vi "Do.vi"(8 "error in (no error)":errorcluster, 10 "Actor in":refnum<class "Actor.lvclass">, 11 "SetInputChannels Msg":refnum<class "SetInputChannels Msg.lvclass">) -> (0 "error out":errorcluster, 2 "Actor out":refnum<class "Actor.lvclass">)   [LabVIEW 2023, in "Multiharp.lvlib" / "SetInputChannels Msg.lvclass"]
doc: "This VI delivers the message to the actor by calling the appropriate method(s) on the actor."
uses:
  SetInputChannels Msg.lvclass
  SetInputChannels Msg.lvclass/SetInputChannels Msg.ctl
  bbf59504-f208-437b-af2f-d262c82c43a6.vi
  Multiharp/Multiharp.lvclass
  <vilib>/ActorFramework/Actor/Actor.lvclass
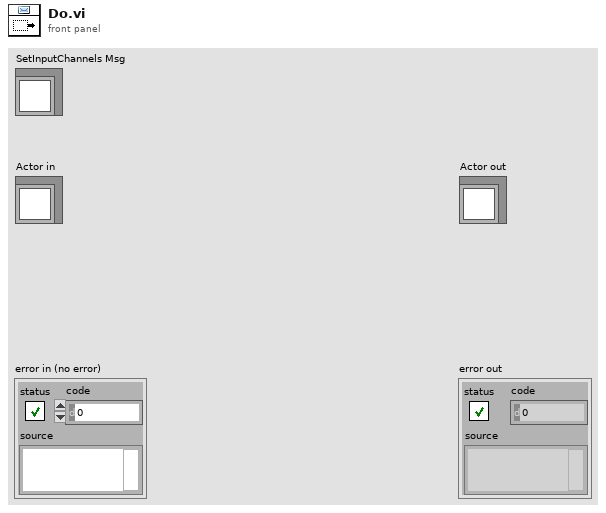
[diagram p1: front panel]
types:
  T1 = typedef "MH_SetInpChanData.ctl" = cluster{"Channel":i32, "Cmds":T2[], "Changed":cluster{"Name":bool, "Enable":bool, "Edge":bool, "Level":bool, "Offset":bool, "UseDeadTime":bool, "DeadTime":bool}}
  T2 = typedef "MH_SetInpChanCmds.ctl" = enum16{"SetInpChanEnable", "SetInpChanOffset", "SetInpChanDeadTime", "SetInpChanTrg"}
  T3 = typedef "MH_InputChannel.ctl" = cluster{"Name":string, "Enable":bool, "Edge":i32, "Level":i32, "Offset":i32, "UseDeadTime":bool, "DeadTime":i32}
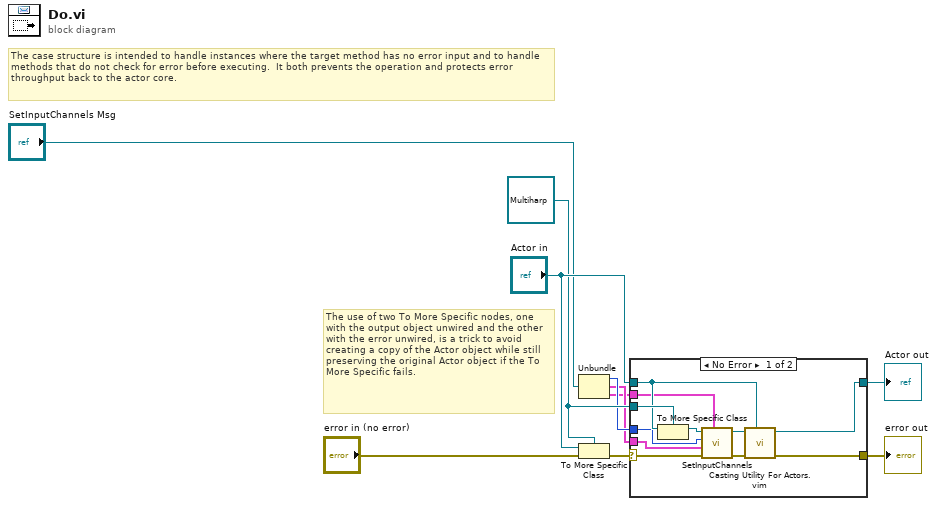
[diagram p0: block diagram]
diagram:
  w5 = refnum<class "Multiharp.lvclass"> refnum ("Actor in")
  # "The use of two To More Specific nodes, one with the output object unwired and the other with the error unwired, is a trick to avoid creating a copy of the Actor object while still preserving the original Actor object if the To More Specific fails."
  # "The case structure is intended to handle instances where the target method has no error input and to handle methods that do not check for error before executing.  It both prevents the operation and protects error throughput back to the actor core."
  n1 = Unbundle("SetInputChannels Msg") -> (w3:i32, w2:T1[], w1:T3[])
  n2 = To More Specific Class(target class=w5, reference="Actor in", error in="error in (no error)") -> (error out=w4:errorcluster)  [unwired: 1 out]
  n3 = case shown="No Error" w4 {
    selector: w4 -> [w21 w23]
    tunnel: [w15 w23] -> w10
    tunnel: [w16 w22] -> w9
    tunnel: "Actor in" -> [w18 w22]
    tunnel: w5 -> [w19 _]
    tunnel: w3 -> [w13 _]
    tunnel: w2 -> [w12 _]
    tunnel: w1 -> [w11 _]
    frame No Error {
      n4 = To More Specific Class(target class=w19, reference=w18) -> (specific class reference=w20:refnum<class "Multiharp.lvclass">)  [unwired: 1 in, 1 out]
      n5 = call-dynamic "SetInputChannels.vi"("Channels"=w11, "error in (no error)"=w21, "SetInpChan"=w12, "features"=w13, "Multiharp in"=w20) -> ("error out"=w14:errorcluster, "Multiharp out"=w17:refnum<class "Multiharp.lvclass">)  [unwired: 5 in]
      n6 = call "Casting Utility For Actors.vim"("type"=w18, "error in (no error)"=w14, "Actor in"=w17) -> ("error out"=w15:errorcluster, "Actor out"=w16:refnum<class "Actor.lvclass">)  [unwired: 7 in]
    }
    frame Error {
      # "If type check fails, pass the original object out again."
    }
  }
  "error out" <- w10
  "Actor out" <- w9
